vi "Finish Scan.vi"(8 "error in (no error)":errorcluster, 11 "Continuous in":refnum<class "Continuous.lvclass">) -> (0 "error out":errorcluster, 3 "Continuous out":refnum<class "Continuous.lvclass">)   [LabVIEW 2015, in "Continuous.lvclass"]
uses:
  Continuous.lvclass
  Instruments/Magnet/Power Supply/Power Supply.lvclass
panel:
  out "persis?":bool caption="Persistent"
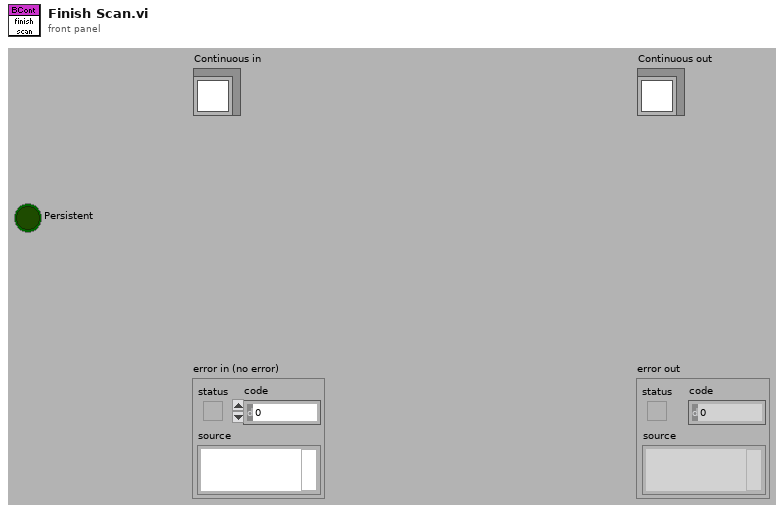
[diagram p1: front panel]
types:
  T1 = typedef "Scanner.lvclass/Range.ctl" = cluster{"xi":dbl, "xf":dbl, "dx":dbl, "Return to...?":bool, "Return to":dbl}
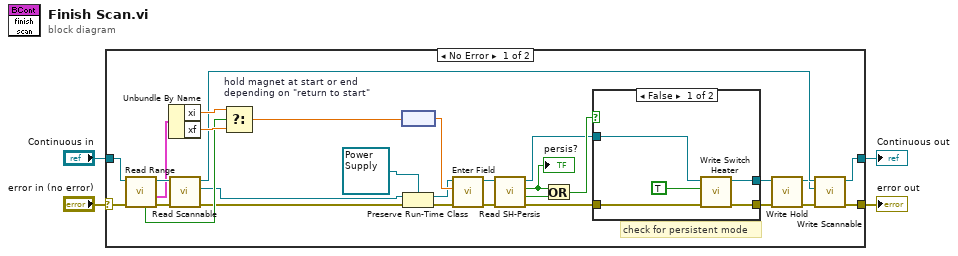
[diagram p0: block diagram]
diagram:
  n1 = case shown="No Error" "error in (no error)" {
    selector: "error in (no error)" -> [w32 w42]
    tunnel: [w7 w42] -> w4
    tunnel: [w26 w41] -> w3
    tunnel: "Continuous in" -> [w31 w41]
    frame No Error {
      # "check for persistent mode"
      n2 = call-dynamic "Read Range.vi"("error in (no error)"=w32, "Scanner.lvclass in"=w31) -> ("error out"=w6:errorcluster, "Range"=w5:T1, "Scanner.lvclass out"=w33:refnum<class "Continuous.lvclass">, "Return to start?"=w28:bool)  [unwired: 6 out]
      n3 = Unbundle By Name(w5) -> ("xi"=w30:dbl, "xf"=w29:dbl)
      n4 = call-dynamic "Read Scannable.vi"("error in (no error)"=w6, "Scanner.lvclass in"=w33) -> ("error out"=w23:errorcluster, "Scannable.lvclass"=w22:refnum<class "Scannable.lvclass">, "Scanner.lvclass out"=w27:refnum<class "Continuous.lvclass">)  [unwired: 7 in]
      n5 = Select "hold magnet at start or end\ndepending on \"return to start\""(t=w30, s=w28, f=w29) -> (s? t:f=w25:dbl)
      n6 = node(w25) -> (w24:dbl[unit])
      n7 = Preserve Run-Time Class(object in=w22, error in=w23, 2:refnum<class "Power Supply.lvclass"> refnum ("Power Supply out")) -> (object out=w21:refnum<class "Power Supply.lvclass">, error out=w20:errorcluster)
      n8 = call-dynamic "Enter Field.vi"("error in (no error)"=w20, "Target field"=w24, "Power Supply in"=w21) -> ("error out"=w9:errorcluster, "Power Supply out"=w8:refnum<class "Power Supply.lvclass">)  [unwired: 7 in]
      n9 = call-dynamic "Read SH-Persis.vi"("error in (no error)"=w9, "Power Supply in"=w8) -> ("error out"=w10:errorcluster, "SHon?"=w17:bool, "pers?"=w16:bool, "Power Supply out"=w15:refnum<class "Power Supply.lvclass">)  [unwired: 4 in, 2 out]
      "persis?" <- w16
      n10 = Or(x=w16, y=w17) -> (x .or. y?=w18:bool)
      n11 = case shown="False" w18 {
        tunnel: w15 -> [w38 w40]
        tunnel: [w37 w40] -> w14
        tunnel: [w36 w39] -> w11
        tunnel: w10 -> [w35 w39]
        frame False {
          n12 = call-dynamic "Write Switch Heater.vi"("error in (no error)"=w35, "Turn SH On?"=TRUE, "Power Supply in"=w38) -> ("error out"=w36:errorcluster, "Power Supply out"=w37:refnum<class "Power Supply.lvclass">)  [unwired: 7 in]
        }
        frame True {
        }
      }
      n13 = call-dynamic "Write Hold.vi"("error in (no error)"=w11, "Power Supply in"=w14) -> ("error out"=w12:errorcluster, "Power Supply out"=w13:refnum<class "Power Supply.lvclass">)  [unwired: 8 in]
      n14 = call-dynamic "Write Scannable.vi"("error in (no error)"=w12, "Scannable.lvclass"=w13, "Scanner.lvclass in"=w27) -> ("error out"=w7:errorcluster, "Scanner.lvclass out"=w26:refnum<class "Continuous.lvclass">)  [unwired: 7 in]
    }
    frame Error {
    }
  }
  "error out" <- w4
  "Continuous out" <- w3
